vi "Set_Text_Argument.vi"(1 "Text":string, 2 "Argument":string, 3 "Argument List In":string[](array[string])) -> (0 "Argument List Out":string[](array[string]))   [LabVIEW 2011]
doc: "This VI sets a textual argument in an argument list. For example, a textual argument of the name \"SomeArgument\" with the value of \"some text\" would be represented by the following string stored in the \"Argument List\" array:\n\nSomeArgument(\"some text\").\n\nThe quotes are necessary to denote a text value. All newline characters should be purged as well, as these will cause problems when saving and loading argument lists from text files."
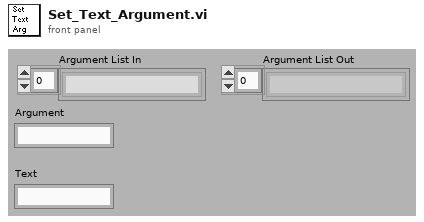
[diagram p1: front panel]
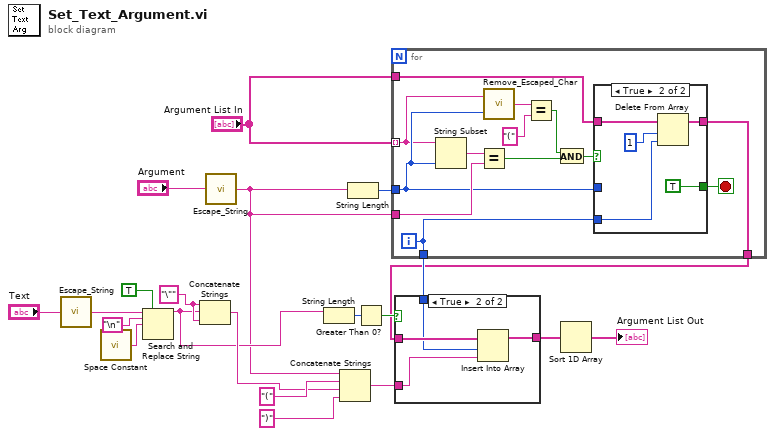
[diagram p0: block diagram]
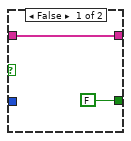
[diagram p3: hidden frame]
diagram:
  w12 = "\"" ("string")
  n1 = call "Escape_String.vi"("Input String"="Text") -> ("Escaped String"=w3:string)
  n2 = call <vilib>:"Space Constant.vi"() -> ("String"=w5:string)
  n3 = Search and Replace String(replace all?=TRUE ("replace all? (F)"), input string=w3, search string="\n", replace string=w5) -> (result string=w8:string)  [unwired: 1 in, 6 out]
  n4 = Concatenate Strings(w12, w8, w12) -> (w11:string)
  n5 = call "Escape_String.vi"("Input String"="Argument") -> ("Escaped String"=w2:string)
  n6 = String Length(string=w8) -> (length=w13:i32)
  n7 = Concatenate Strings(w2, "(" ("string"), w11, ")" ("string")) -> (w16:string)
  n8 = String Length(string=w2) -> (length=w21:i32)
  n9 = Greater Than 0?(x=w13) -> (x > 0?=w20:bool)
  n10 = for {
    tunnel: "Argument List In" -> [w23] mode=indexing
    tunnel: w21 -> [w24]
    tunnel: w2 -> [w33]
    tunnel: "Argument List In" -> [w31]
    tunnel: [w30] -> w19
    tunnel: [w29] -> w14
    i -> [w30]
    stop <- w32 stop-if-true
    n11 = String Subset(string=w23, length (rest)=w24) -> (substring=w34:string)  [unwired: 1 out]
    n12 = Equal?(x=w34, y=w33) -> (x = y?=w28:bool)
    n13 = call "Remove_Escaped_Char.vi"("Offset"=w24, "Input String"=w23) -> ("Output String"=w22:string)
    n14 = Equal?(x=w22, y="(") -> (x = y?=w26:bool)
    n15 = And(x=w26, y=w28) -> (x .and. y?=w25:bool)
    n16 = case shown="True" w25 {
      tunnel: w24 -> [_ _]
      tunnel: [FALSE TRUE] -> w32
      tunnel: w30 -> [_ w40]
      tunnel: w31 -> [w35 w39]
      tunnel: [w35 w37] -> w29
      frame False {
      }
      frame True {
        n17 = Delete From Array(array=w39, length=1, index=w40) -> (array with subset deleted=w37:string[])  [unwired: 1 out]
      }
    }
  }
  n18 = case shown="True" w20 {
    tunnel: w14 -> [w42 w46]
    tunnel: w19 -> [_ w45]
    tunnel: w16 -> [_ w44]
    tunnel: [w42 w43] -> w15
    frame False {
    }
    frame True {
      n19 = Insert Into Array(array=w46, index=w45, new element=w44) -> (w43:string[])
    }
  }
  n20 = Sort 1D Array(array=w15) -> (sorted array=→"Argument List Out":string[])
